vi "transBendingModeCoorSys.vi"(8 "error in (no error)":errorcluster, 9 "Mirror DOF (um)":dbl[](array[numeric]), 10 "Mirror":enum16{"M1M3", "M2"}(ring), 11 "SubSysAdap in":refnum<class "SubSysAdap.lvclass">) -> (0 "error out":errorcluster, 2 "Transformed Mirror DOF (um)":dbl[](array[numeric]), 3 "SubSysAdap out":refnum<class "SubSysAdap.lvclass">)   [LabVIEW 2016, in "SubSysAdap.lvclass"]
doc: "Transform the bending mode (degree of freedom, DOF) from Bo's FEA model to Chris's FEA model. This function should be removed in the final once there is a unified FEA model."
uses:
  SubSysAdap.lvclass
  SubSysAdap.lvclass/SubSysAdap.ctl
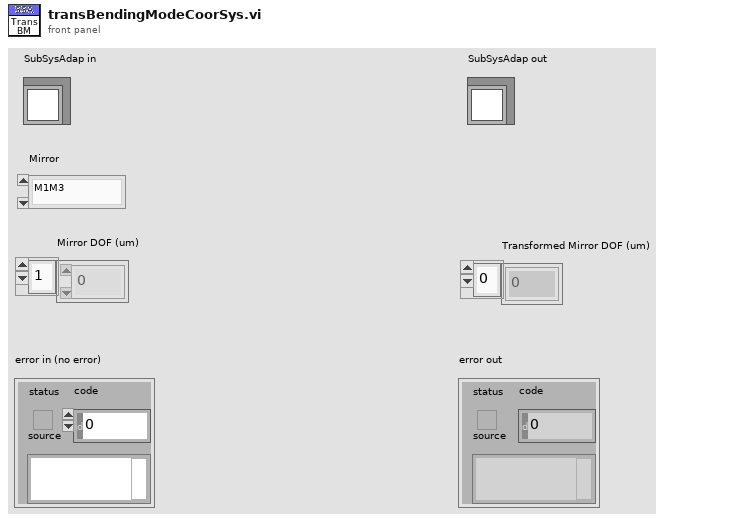
[diagram p1: front panel]
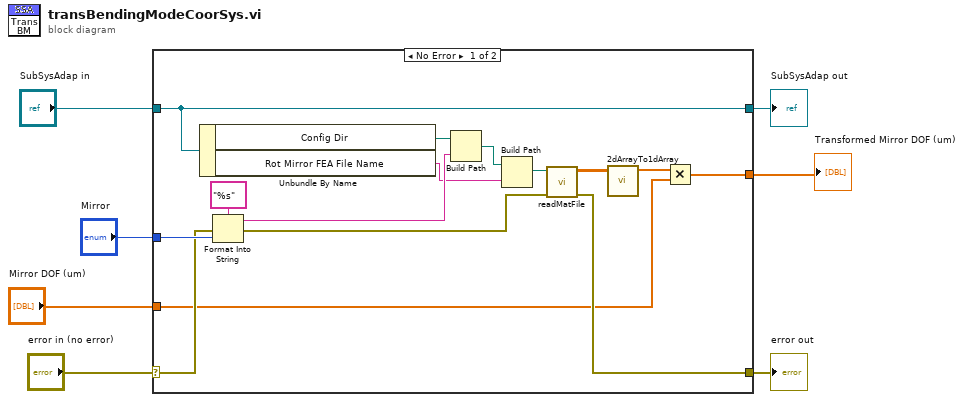
[diagram p0: block diagram]
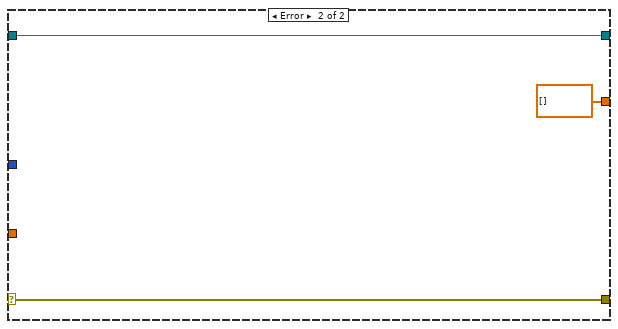
[diagram p2: hidden frame]
diagram:
  n1 = case shown="No Error" "error in (no error)" {
    selector: "error in (no error)" -> [w11 w25]
    tunnel: [w10 w25] -> w6
    tunnel: [w13 w24] -> w4
    tunnel: "SubSysAdap in" -> [w13 w24]
    tunnel: "Mirror" -> [w12 _]
    tunnel: "Mirror DOF (um)" -> [w9 _]
    tunnel: [w8 dbl[] []] -> w1
    frame No Error {
      n2 = Unbundle By Name(w13) -> ("Config Dir"=w21:path, "Rot Mirror FEA File Name"=w18:string)
      n3 = Format Into String(format string="%s", error in=w11, w12) -> (resulting string=w19:string, error out=w16:errorcluster)  [unwired: 1 in]
      n4 = Build Path(base path=w21, name or relative path=w19) -> (appended path=w20:path)
      n5 = Build Path(base path=w20, name or relative path=w18) -> (appended path=w17:path)
      n6 = call "readMatFile.vi"("error in (no error)"=w16, "Path"=w17) -> ("error out"=w10:errorcluster, "Matrix"=w15:dbl[][])  [unwired: 8 in]
      n7 = call "2dArrayTo1dArray.vi"("2D Array"=w15) -> ("1D Array"=w14:dbl[])  [unwired: 10 in]
      n8 = Multiply(x=w14, y=w9) -> (x*y=w8:dbl[])
    }
    frame Error {
    }
  }
  "error out" <- w6
  "SubSysAdap out" <- w4
  "Transformed Mirror DOF (um)" <- w1
